vi "GetReferenceDataType.vi"(8 "error in":errorcluster, 10 "Channel Number":i32=1 min=1 max=52, 11 "VISA resource name":refnum<visa-resource-name>) -> (0 "error out":errorcluster, 2 "Reference Data Type":string, 3 "VISA resource name out":refnum<visa-resource-name>)   [LabVIEW 2023, in "Thermotron 8800.lvlib"]
doc: "DREF\nCommand name: Send reference data type\nCommand type: System status\nDescription: The 8800 sends an integer representing the channel’s reference channel data type.\nData type codes:\n0 Unused\n1 Temperature\n2 RH wet bulb/dry bulb\n3 RH linear\n4 RH temperature compensated\n5 Linear\n6 Altitude (kilofeet)\n7 Vibration\n8 Scaled linear\n9 Altitude linear (torr)\nFor example, assume channel 2 is an RH temperature-compensated channel\nreferencing channel 1, which is a temperature channel. Sending DREF2? will return a 1\n(temperature), the data type of channel 2’s reference channel.\nSyntax: DREFn?\nWhere n is a channel number (1 through 52).\n1 through 8 Process variable channels\n9 through 12 Unused\n13 through 52 Monitor channels (1 through 40).\nData type: Integer\nQuery example: DREF2?\n8800 response: 1 (The data type of channel 2’s reference channel is temperature.)"
uses:
  Thermotron 8800.lvlib
panel:
  # "Data type codes:\n0 Unused\n1 Temperature\n2 RH wet bulb/dry bulb\n3 RH linear\n4 RH temperature compensated\n5 Linear\n6 Altitude (kilofeet)\n7 Vibration\n8 Scaled linear\n9 Altitude linear (torr)"
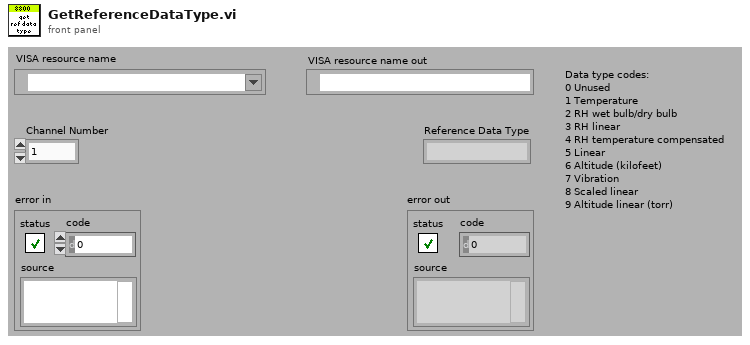
[diagram p1: front panel]
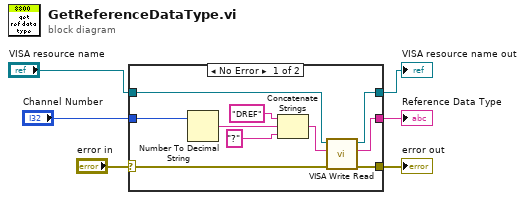
[diagram p0: block diagram]
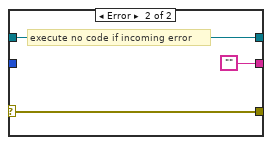
[diagram p2: hidden frame]
diagram:
  n1 = case shown="No Error" "error in" {
    selector: "error in" -> [w14 w18]
    tunnel: [w11 w18] -> w5
    tunnel: [w12 w19] -> w4
    tunnel: "VISA resource name" -> [w13 w19]
    tunnel: [w10 ""] -> w2
    tunnel: "Channel Number" -> [w9 _]
    frame No Error {
      n2 = Number To Decimal String(number=w9) -> (decimal integer string=w7:string)  [unwired: 1 in]
      n3 = Concatenate Strings("DREF" ("8800 Command"), w7, "?" ("8800 Command")) -> (w16:string)
      n4 = call "VISA Write Read.vi"("error in (no error)"=w14, "8800 Command"=w16, "VISA Refnum in"=w13) -> ("error out"=w11:errorcluster, "read buffer"=w10:string, "VISA Refnum out"=w12:refnum<visa-resource-name>)  [unwired: 6 in]
    }
    frame Error {
      # "execute no code if incoming error"
    }
  }
  "VISA resource name out" <- w4
  "error out" <- w5
  "Reference Data Type" <- w2
